vi "frequency_to_rpm.vi"(7 "Number of Stickers":i64, 11 "Pulse Frequency [Hz]":dbl) -> (3 "Spin [RPM]":dbl)   [LabVIEW 2025, in "LabJackEKG.lvlib"]
uses:
  LabJackEKG.lvlib
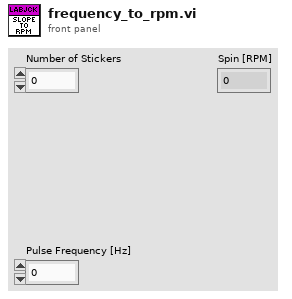
[diagram p1: front panel]
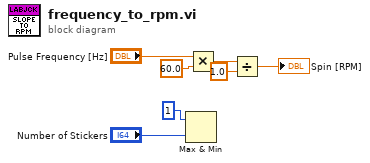
[diagram p0: block diagram]
diagram:
  n1 = Max & Min(x=i64 1, y="Number of Stickers") -> ()  [unwired: 2 out]
  n2 = Multiply(x="Pulse Frequency [Hz]", y=60.0) -> (x*y=w3:dbl)
  n3 = Divide(x=w3, y=1.0) -> (x/y=→"Spin [RPM]":dbl)
